vi "fgv_rplidar_config.vi"(7 "cmd":enum16{"read", "write"}(ring), 8 "error in":errorcluster, 11 "RPLidar cfg":T1={"port"="COM6", "dt"=6, "update n"=8, "speed"=272, "rate "=256000} {"speed" scale=100.0..1000.0}) -> (0 "error out":errorcluster, 3 "RPLidar cfg out":T1={"port"="COM6", "dt"=6, "update n"=8, "speed"=272, "rate "=256000} {"speed" scale=100.0..1000.0})   [LabVIEW 2019]
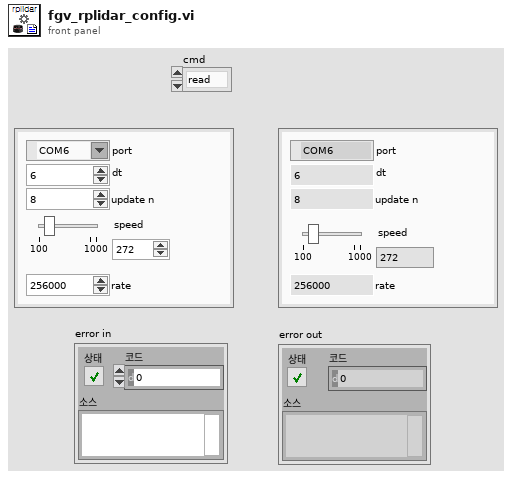
[diagram p1: front panel]
types:
  T1 = cluster{"port":refnum<visa-resource-name>, "dt":u32, "update n":u8, "speed":u16, "rate ":u32}
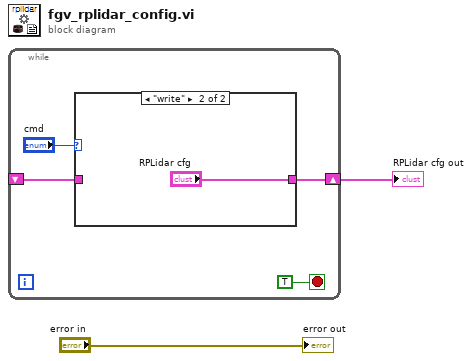
[diagram p0: block diagram]
diagram:
  n1 = while {
    shift-right: [w4] -> w2
    shift-left: _ -> [w3]
    stop <- TRUE stop-if-true
    n2 = case shown="\"write\"" "cmd" {
      tunnel: [w7 "RPLidar cfg"] -> w4
      tunnel: w3 -> [w7 _]
      frame "read", Default {
      }
      frame "write" {
      }
    }
  }
  "RPLidar cfg out" <- w2
  "error out" <- "error in"
